vi "setWheelData_ShootDualTalonSRX.vi"(6 "Time":T2, 7 "Distance Type":T1, 9 "Enc Edges / Rev":dbl=1440.0 format="%.4f", 11 "Wheel Radius In":dbl=3.0 format="%.4f") -> (0 "VelUnits/Count in 0.1":dbl format="%.4f", 1 "Count/VelUnits In 0.1 SEC":dbl format="%.4f", 2 "Dist/Count":dbl format="%.4f", 3 "Count/Dist":dbl format="%.4f", 4 "Units":string)   [LabVIEW 2019, in "ShootDualTalonSRX_Motor_Pair.lvlib"]
uses:
  ShootDualTalonSRX_Motor_Pair.lvlib
  Time_Units_Control.ctl
  Dist_Type.ctl
  globals_ShootDualTalonSRX.vi
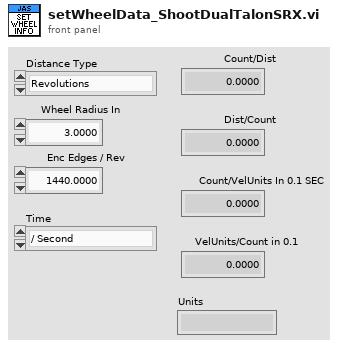
[diagram p1: front panel]
types:
  T1 = typedef "ShootDualTalonSRX_Motor_Pair.lvlib/Dist_Type.ctl" = enum16{"Revolutions", "Feet"}
  T2 = typedef "ShootDualTalonSRX_Motor_Pair.lvlib/Time_Units_Control.ctl" = enum16{"/ Second", "/ Minute"}
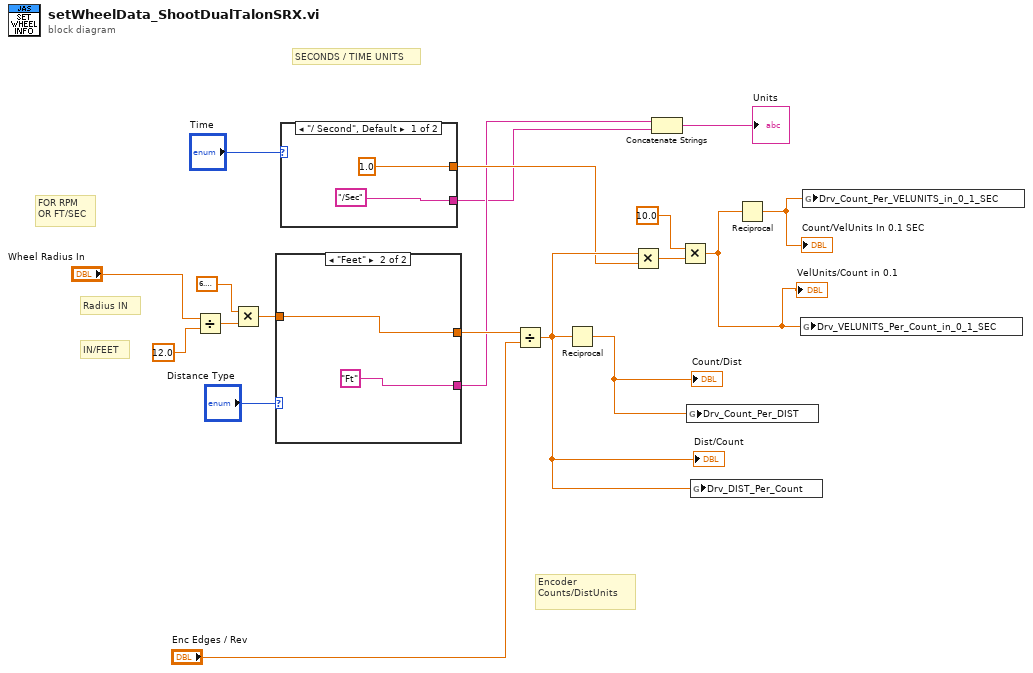
[diagram p0: block diagram]
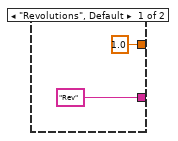
[diagram p2: hidden frame]
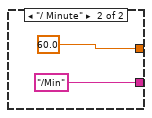
[diagram p3: hidden frame]
diagram:
  # "Encoder\nCounts/DistUnits"
  # "SECONDS / TIME UNITS"
  # "FOR RPM\nOR FT/SEC"
  # "IN/FEET"
  # "Radius IN"
  n1 = Divide(x="Wheel Radius In", y=12.0) -> (x/y=w15:dbl)
  n2 = Multiply(x=6.283185307179586, y=w15) -> (x*y=w10:dbl)
  n3 = case shown="\"Feet\"" "Distance Type" {
    tunnel: w10 -> [_ w23]
    tunnel: [1.0 w23] -> w9
    tunnel: ["Rev" "Ft"] -> w5
    frame "Revolutions", Default {
    }
    frame "Feet" {
    }
  }
  n4 = case shown="\"/ Second\", Default" "Time" {
    tunnel: [1.0 60.0] -> w6
    tunnel: ["/Sec" "/Min"] -> w4
    frame "/ Second", Default {
    }
    frame "/ Minute" {
    }
  }
  n5 = Divide(x=w9, y="Enc Edges / Rev") -> (x/y=w7:dbl)
  "Dist/Count" <- w7
  n6 = Reciprocal(x=w7) -> (1/x=w19:dbl)
  "Count/Dist" <- w19
  n7 = Multiply(x=w7, y=w6) -> (x*y=w8:dbl)
  n8 = Concatenate Strings(w5, w4) -> (→"Units":string)
  n9 = Multiply(x=10.0 ("y"), y=w8) -> (x*y=w2:dbl)
  "VelUnits/Count in 0.1" <- w2
  n10 = global write "globals_ShootDualTalonSRX.vi" "Drv_Count_Per_DIST"(w19) -> ()
  n11 = global write "globals_ShootDualTalonSRX.vi" "Drv_DIST_Per_Count"(w7) -> ()
  n12 = Reciprocal(x=w2) -> (1/x=w1:dbl)
  "Count/VelUnits In 0.1 SEC" <- w1
  n13 = global write "globals_ShootDualTalonSRX.vi" "Drv_VELUNITS_Per_Count_in_0_1_SEC"(w2) -> ()
  n14 = global write "globals_ShootDualTalonSRX.vi" "Drv_Count_Per_VELUNITS_in_0_1_SEC"(w1) -> ()
